vi "Analog Input (Host).vi"() -> ()   [LabVIEW 2016]
uses:
  <vilib>/FPGAPlugInAG/PXIe-7847R/niLvFpga_Open_PXIe-7847R.vi
  <vilib>/rvi/interface/common/dynamic/niFpgaDynamicAddResources.vi
  <vilib>/Utility/error.llb/Error Cluster From Error Code.vi
  <vilib>/rvi/errors/niLvFpgaAdjustHostInterfaceError.vi
  <vilib>/rvi/interface/nirviOpenFPGA/nirviOpenFPGA.xnode
  FPGA_Bitfiles/AnalogInput-FPGA-test.lvbitx
  Analog Input.vi
  <vilib>/rvi/interface/nirviReadWriteControl/nirviReadWriteControl.xnode
  NiFpgaLv.dll
  <vilib>/rvi/interface/Simulation/niFpgaSimulationCallBeginRW.vi
panel:
  in  "stop":bool
  out "Waveform Chart":cluster{dbl, dbl, dbl, dbl, dbl, dbl}(graph)
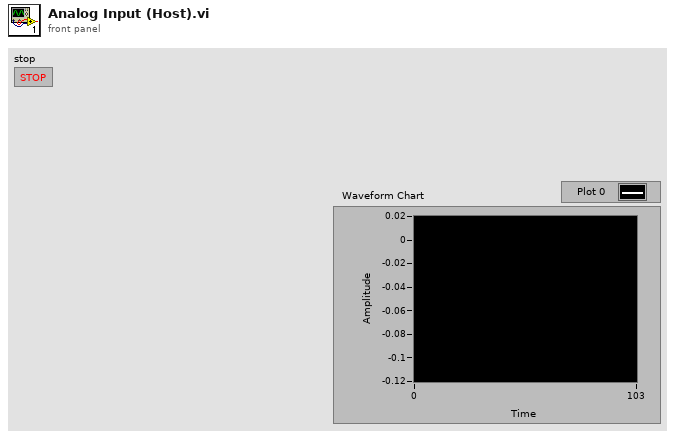
[diagram p1: front panel]
types:
  T1 = cluster{"Connector0/AI0":fxp<+/-,27,5>, "Connector0/AI1":fxp<+/-,27,5>, "Connector0/AI2":fxp<+/-,27,5>, "Connector0/AI3":fxp<+/-,27,5>, "Connector0/AI4":fxp<+/-,27,5>, "Connector0/AI5":fxp<+/-,27,5>}
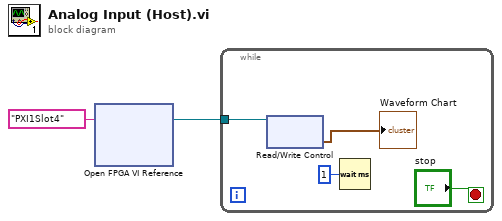
[diagram p0: block diagram]
diagram:
  n1 = xnode "Open FPGA VI Reference"("resource name"=tag "PXI1Slot4") -> ("FPGA VI Reference Out"=w2:refnum<k20>)  [unwired: 1 in, 1 out]
  n2 = while {
    tunnel: w2 -> [w6]
    stop <- "stop" stop-if-true
    n3 = xnode "Read/Write Control"("FPGA VI Reference In"=w6) -> ("AI Data"=→"Waveform Chart":T1)  [unwired: 1 in, 2 out]
    n4 = Wait (ms)(milliseconds to wait=u32 1) -> ()  [unwired: 1 out]
  }
